vi "JSON text to Variant.vi"(6 "LVClass Serializer":refnum<class "JSONtext LVClass Serializer.lvclass">, 8 "error in (no error)":errorcluster, 9 "Data Type":variant, 10 "Offset":i32, 11 "JSON":string) -> (0 "error out":errorcluster, 1 "Variant out":variant)   [LabVIEW 2020, in "JSONtext.lvlib"]
doc: "Convert JSON to the Data Type entered, which may be a cluster or array."
uses:
  <vilib>/JDP Science/JSONtext/JSONtext.lvlib
  <vilib>/JDP Science/JSONtext/LVClass Serializer/JSONtext LVClass Serializer.lvclass
  <vilib>/Utility/Data Type/Type Definitions/Data Type.ctl
  <vilib>/JDP Science/JSONtext/support/Get String.vi
  <vilib>/JDP Science/JSONtext/support/Get Timestamp.vi
  <vilib>/JDP Science/JSONtext/support/Get I32.vi
  <vilib>/JDP Science/JSONtext/support/Coerce I32 to Variant Intger.vi
  <vilib>/JDP Science/JSONtext/support/Get I64.vi
  <vilib>/JDP Science/JSONtext/support/Get U32.vi
  <vilib>/JDP Science/JSONtext/support/Coerce U32 to Variant Intger.vi
  <vilib>/JDP Science/JSONtext/support/Get U64.vi
  <vilib>/JDP Science/JSONtext/support/Get Boolean.vi
  <vilib>/JDP Science/JSONtext/support/Get DBL.vi
  <vilib>/JDP Science/JSONtext/support/Get SGL.vi
  <vilib>/JDP Science/JSONtext/support/Unescape JSON string.vi
  <vilib>/JDP Science/JSONtext/support/quote and escape json string 2.vi
  <vilib>/JDP Science/JSONtext/support/Commas Needed.vi
  <vilib>/JDP Science/JSONtext/Parsing/Advance past whitespace and comma.vi
  <vilib>/JDP Science/JSONtext/Parsing/Advance past next JSON Value (inlined COPY).vi
  <vilib>/JDP Science/JSONtext/Parsing/Advance past Item Name.vi
  <vilib>/JDP Science/JSONtext/Base64/base64url Decode.vi
  <vilib>/JDP Science/JSONtext/Parsing/Advance past Line Ending.vi
  <vilib>/JDP Science/JSONtext/Parsing/Advance past String.vi
  <vilib>/JDP Science/JSONtext/support/Get Number Text.vi
  <vilib>/JDP Science/JSONtext/Parsing/NaN or null to Integer ERROR.vi
  <vilib>/JDP Science/JSONtext/Parsing/Advance past Number.vi
  <vilib>/Utility/error.llb/Error Cluster From Error Code.vi
  <vilib>/Utility/Data Type/Get Refnum Information.vi
  <vilib>/JDP Science/JSONtext/support/Error Cluster From Code.vi
  <vilib>/JDP Science/JDP Science Common Utilities/Timestamp/Text to Timestamp.vi
  <vilib>/Utility/Data Type/Get Numeric Information.vi
  <vilib>/JDP Science/JSONtext/Parsing/Advance past Object.vi
  <vilib>/JDP Science/JSONtext/Parsing/Parsing Error.vi
  <vilib>/Utility/Data Type/NI_Data Type.lvlib
  <vilib>/JDP Science/JDP Science Common Utilities/JDP Utility.lvlib
  <vilib>/JDP Science/JSONtext/support/Set Map/SetMap.lvlib
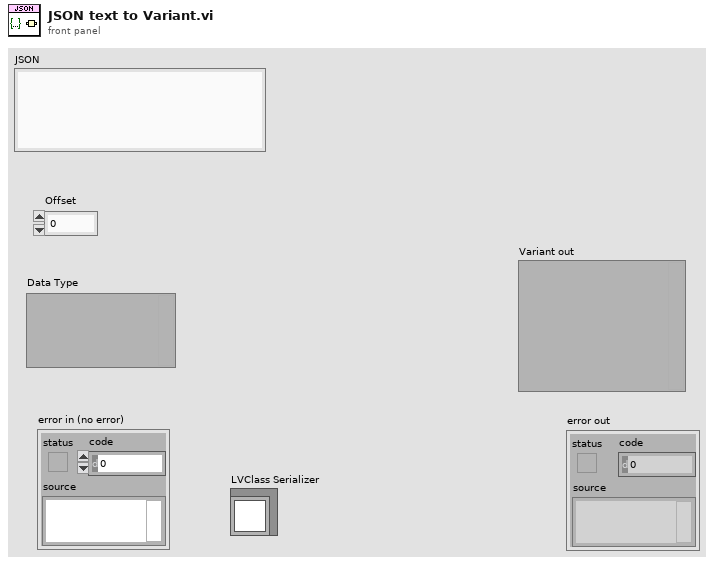
[diagram p1: front panel]
types:
  T1 = typedef "NI_Data Type.lvlib/Data Type.ctl" = enum8{"Invalid Type", "Void", "I8", "I16", "I32", "I64", "U8", "U16", "U32", "U64", "Single Float", "Double Float", "Extended Float", "Single Complex", "Double Complex", "Extended Complex", "Enum U8", "Enum U16", "Enum U32", "Enum U64", "Single Float With Unit", "Double Float With Unit", "Extended Float With Unit", "Single Complex with Unit", "Double Complex with Unit", "Extended Complex with Unit", "Boolean", "String", "Path", "Picture", "Tag", "Array", "Cluster", "Variant", "LV Variant", "Waveform", "Timestamp", "Digital Waveform", "Digital Data", "ExpressData", "Refnum", "External Data", "VI", "Poly VI", "LabVIEW Class Instance", "Fixed Point", "Set Collection", "Map Collection"}
  T2 = typedef "JSONtext.lvlib/Parsing State.ctl" = enum16{"Parser Error", "Object", "Array", "String", "Number/Other", "Leading Whitespace", "Object end", "Array end", "Value end"}
  T3 = typedef "JSONtext.lvlib/Tag Type.ctl" = enum16{"No Tag", "<JSON>", "<JOBJ>"}
  T4 = typedef "JSONtext.lvlib/JSON Value Type.ctl" = enum16{"Not a JSON Value", "JSON Object", "JSON Array", "String", "Number", "true", "false", "null"}
  T5 = typedef "JSONtext.lvlib/Found Items.ctl" = cluster{"Item offset":i32, "Offset past Item":i32, "Name offset":i32, "Offset past Name":i32, "Found":bool, "Item Type":T2, "Item Index":i32, "Start Offset":i32, "Comma Needed For Insert":T6}
  T6 = typedef "JSONtext.lvlib/Comma Needed for Insert.ctl" = enum8{"False", "True", "Following"}
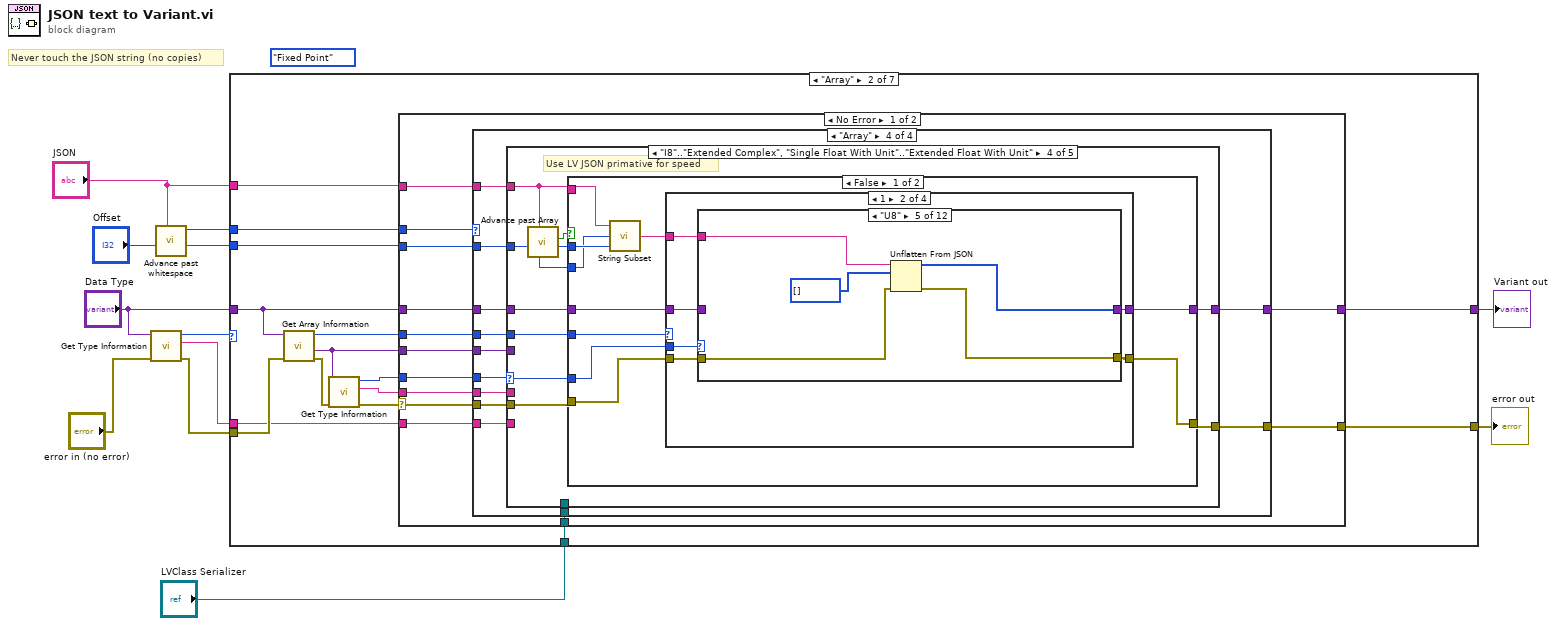
[diagram p0: block diagram]
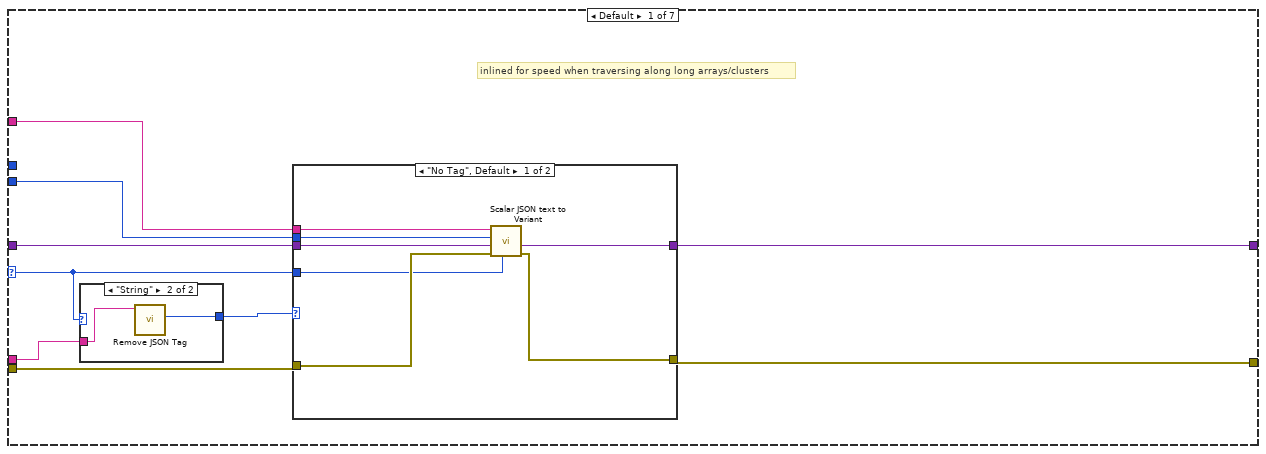
[diagram p2: hidden frame]
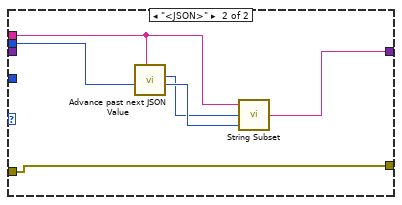
[diagram p3: hidden frame]
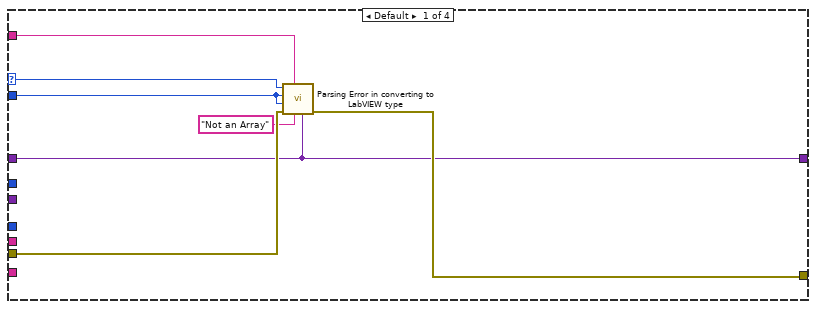
[diagram p5: hidden frame]
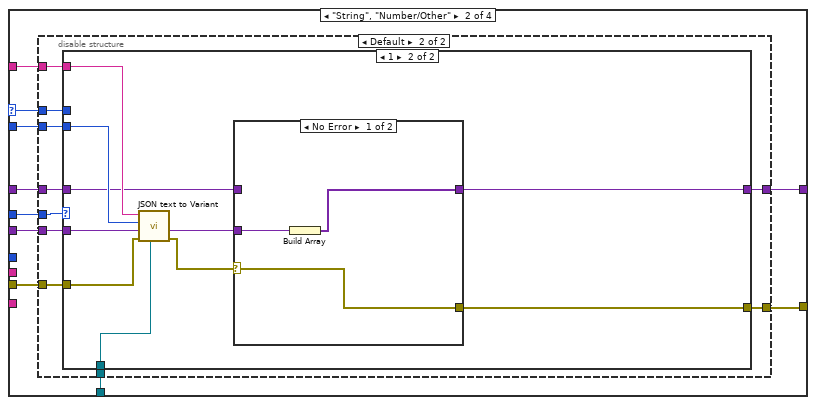
[diagram p6: hidden frame]
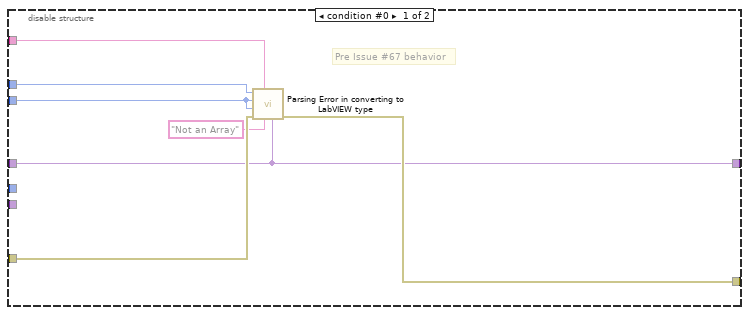
[diagram p7: hidden frame]
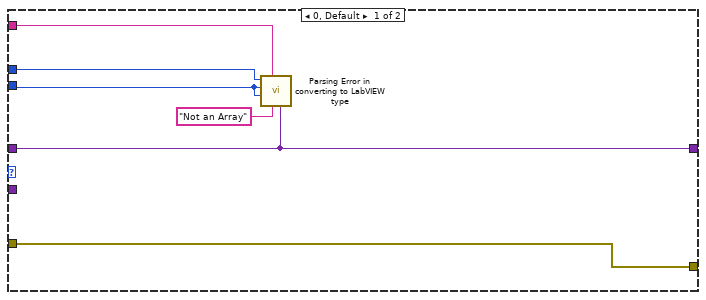
[diagram p8: hidden frame]
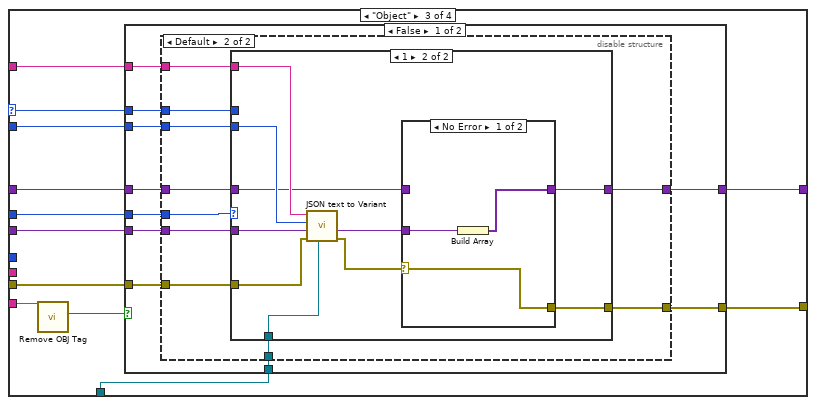
[diagram p10: hidden frame]
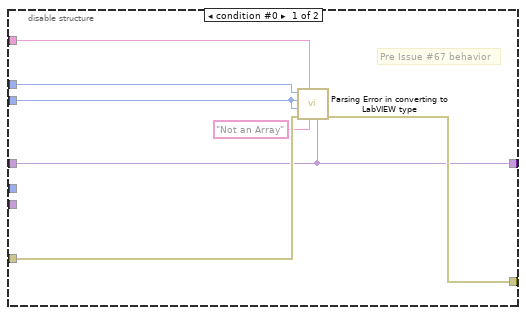
[diagram p11: hidden frame]
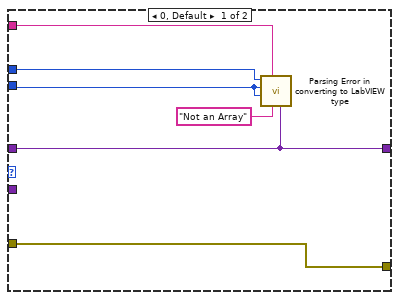
[diagram p12: hidden frame]
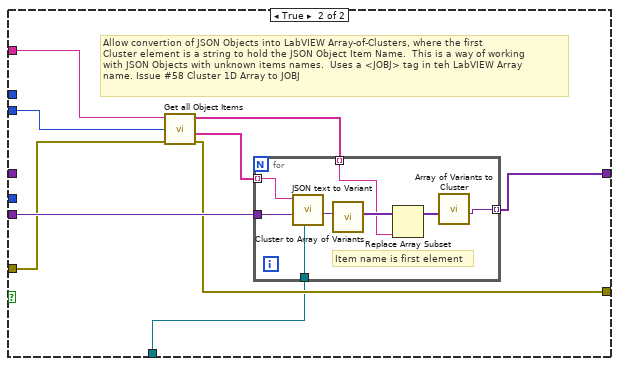
[diagram p14: hidden frame]
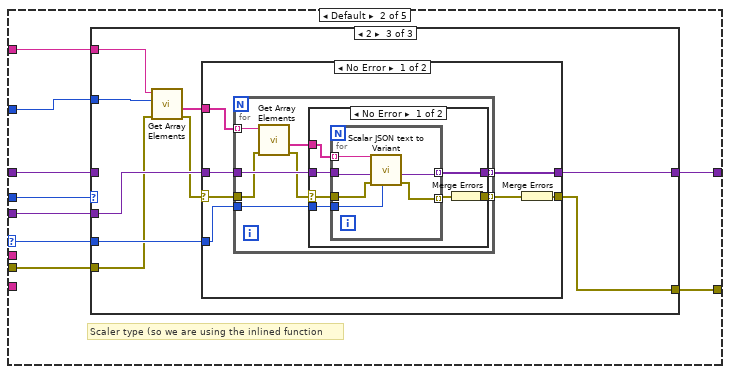
[diagram p16: hidden frame]
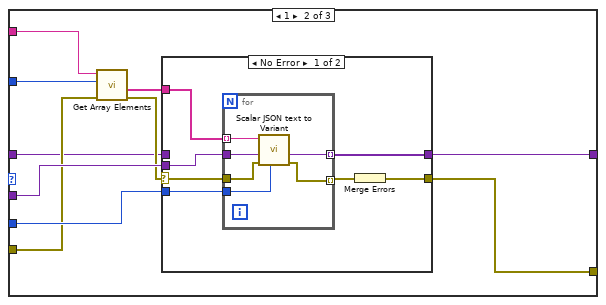
[diagram p18: hidden frame]
diagram:
  (unwired) Data_Type."Fixed Point" ("Type")
  # "Never touch the JSON string (no copies)"
  n1 = call <vilib>:"Get Type Information.vi"("error in (no error)"="error in (no error)", "variant"="Data Type") -> ("error out"=w8:errorcluster, "name"=w2:string, "type"=w12:T1)  [unwired: 5 in, 2 out]
  n2 = call <vilib>:"Advance past whitespace.vi"("JSON"="JSON", "Offset"="Offset") -> ("Offset of first non-whitespace"=w5:i32, "Parser State"=w3:T2)  [unwired: 7 in, 1 out]
  n3 = case shown="\"Array\"" w12 {
    selector: w12 -> [w14 _ _ _ _ _ w916]
    tunnel: "Data Type" -> [w21 w44 w676 w685 w885 w896 w918]
    tunnel: "JSON" -> [w19 w42 w669 w681 w880 w897 w917]
    tunnel: [w16 w48 w666 w683 w877 w890 w912] -> w9
    tunnel: w8 -> [w17 w51 w675 w684 w884 w894 w913]
    tunnel: w5 -> [w18 w40 w668 w682 w879 w889 w915]
    tunnel: [w20 w47 w659 w678 w882 w891 w914] -> w7
    tunnel: w3 -> [_ w38 _ _ _ _ _]
    tunnel: w2 -> [w15 w41 _ _ _ _ _]
    tunnel: "LVClass Serializer" -> [_ w37 w658 w677 w875 w888 w911]
    frame Default {
      # "inlined for speed when traversing along long arrays/clusters"
      n4 = case shown="\"String\"" w14 {
        tunnel: w15 -> [_ w36]
        tunnel: [_ w35] -> w13
        frame "Invalid Type", Default {
        }
        frame "String" {
          n5 = call <vilib>:"Remove JSON Tag.vi"("Name"=w36) -> ("Tag"=w35:T3)  [unwired: 9 in, 1 out]
        }
      }
      n6 = case shown="\"No Tag\", Default" w13 {
        tunnel: w21 -> [w28 _]
        tunnel: [w27 w30] -> w20
        tunnel: w19 -> [w26 w31]
        tunnel: w18 -> [w25 w34]
        tunnel: w17 -> [w24 w29]
        tunnel: [w23 w29] -> w16
        tunnel: w14 -> [w22 _]
        frame "No Tag", Default {
          n7 = call <vilib>:"Scalar JSON text to Variant.vi"("Type"=w22, "error in (no error)"=w24, "Variant (Data Type)"=w28, "Offset"=w25, "JSON"=w26) -> ("error out"=w23:errorcluster, "Variant out"=w27:variant)  [unwired: 5 in]
        }
        frame "<JSON>" {
          n8 = call <vilib>:"Advance past next JSON Value.vi"("JSON"=w31, "Offset"=w34) -> ("Offset out"=w33:i32, "Value start"=w32:i32)  [unwired: 7 in, 1 out]
          n9 = call <vilib>:"String Subset.vi"("Offset past End"=w33, "Start offset"=w32, "JSON"=w31) -> ("substring"=w30:string)  [unwired: 2 in]
        }
      }
    }
    frame "Array" {
      n10 = call <vilib>:"Get Array Information.vi"("error in (no error)"=w51, "variant"=w44) -> ("error out"=w50:errorcluster, "array element data type"=w43:variant, "number of dimensions"=w45:i32)  [unwired: 6 in, 1 out]
      n11 = call <vilib>:"Get Type Information.vi"("error in (no error)"=w50, "variant"=w43) -> ("error out"=w49:errorcluster, "name"=w39:string, "type"=w46:T1)  [unwired: 5 in, 2 out]
      n12 = case shown="No Error" w49 {
        selector: w49 -> [w64 w657]
        tunnel: [w63 w657] -> w48
        tunnel: [w62 w656] -> w47
        tunnel: w46 -> [w61 _]
        tunnel: w45 -> [w60 _]
        tunnel: w44 -> [w59 w656]
        tunnel: w43 -> [w58 _]
        tunnel: w42 -> [w57 _]
        tunnel: w41 -> [w56 _]
        tunnel: w40 -> [w55 _]
        tunnel: w39 -> [w54 _]
        tunnel: w38 -> [w53 _]
        tunnel: w37 -> [w52 _]
        frame No Error {
          n13 = case shown="\"Array\"" w53 {
            selector: w53 -> [w69 w79 w129 _]
            tunnel: w64 -> [w68 w78 w128 w208]
            tunnel: [w67 w77 w127 w207] -> w63
            tunnel: [w66 w74 w124 w206] -> w62
            tunnel: w61 -> [_ _ _ w205]
            tunnel: w60 -> [_ w73 w123 w204]
            tunnel: w59 -> [w66 w76 w126 w203]
            tunnel: w58 -> [_ w75 w125 w202]
            tunnel: w57 -> [w71 w81 w131 w201]
            tunnel: w56 -> [_ _ w121 w200]
            tunnel: w55 -> [w70 w80 w130 w199]
            tunnel: w54 -> [_ _ _ w198]
            tunnel: w52 -> [_ w72 w122 w197]
            frame Default {
              n14 = call <vilib>:"Parsing Error in converting to LabVIEW type.vi"("LV Type"=w66, "initial string"="Not an Array", "JSON"=w71, "error in (no error)"=w68, "Offset past match"=w70, "Value start"=w70, "State"=w69) -> ("error out"=w67:errorcluster)  [unwired: 4 in]
            }
            frame "String", "Number/Other" {
              n15 = disable-structure shown="Default" {
                disable-tunnel: w81 -> [w88 w97]
                disable-tunnel: w80 -> [w87 w96]
                disable-tunnel: w79 -> [w86 w90]
                disable-tunnel: w78 -> [w85 w95]
                disable-tunnel: [w84 w92] -> w77
                disable-tunnel: w76 -> [w82 w93]
                disable-tunnel: w75 -> [_ w98]
                disable-tunnel: [w82 w94] -> w74
                disable-tunnel: w73 -> [_ w91]
                disable-tunnel: w72 -> [_ w89]
                frame condition #0 {
                  # "Pre Issue #67 behavior"
                  n16 = call <vilib>:"Parsing Error in converting to LabVIEW type.vi"("LV Type"=w82, "initial string"="Not an Array", "JSON"=w88, "error in (no error)"=w85, "Offset past match"=w87, "Value start"=w87, "State"=w86) -> ("error out"=w84:errorcluster)  [unwired: 4 in]
                }
                frame condition #1 (active) {
                  n17 = case shown="1" w91 {
                    tunnel: w98 -> [_ w114]
                    tunnel: w97 -> [w103 w113]
                    tunnel: w96 -> [w101 w112]
                    tunnel: w95 -> [w99 w110]
                    tunnel: [w100 w108] -> w94
                    tunnel: w93 -> [w100 w107]
                    tunnel: [w99 w106] -> w92
                    tunnel: w90 -> [w102 _]
                    tunnel: w89 -> [_ w105]
                    frame 0, Default {
                      n18 = call <vilib>:"Parsing Error in converting to LabVIEW type.vi"("LV Type"=w100, "initial string"="Not an Array", "JSON"=w103, "Offset past match"=w101, "Value start"=w101, "State"=w102) -> ()  [unwired: 5 in, 1 out]
                    }
                    frame 1 {
                      n19 = call <vilib>:"JSON text to Variant.vi"("LVClass Serializer"=w105, "error in (no error)"=w110, "Data Type"=w114, "Offset"=w112, "JSON"=w113) -> ("error out"=w109:errorcluster, "Variant out"=w111:variant)  [unwired: 5 in]
                      n20 = case shown="No Error" w109 {
                        selector: w109 -> [w115 w118]
                        tunnel: w111 -> [w117 _]
                        tunnel: [w116 w119] -> w108
                        tunnel: w107 -> [_ w119]
                        tunnel: [w115 w118] -> w106
                        frame No Error {
                          n21 = Build Array(w117) -> (w116:variant[])
                        }
                        frame Error {
                        }
                      }
                    }
                  }
                }
              }
            }
            frame "Object" {
              n22 = call <vilib>:"Remove OBJ Tag.vi"("Name"=w121) -> ("tagged as Item Name in JSON Objects"=w120:bool)  [unwired: 9 in, 1 out]
              n23 = case shown="False" w120 {
                tunnel: w131 -> [w141 w186]
                tunnel: w130 -> [w140 w180]
                tunnel: w129 -> [w139 _]
                tunnel: w128 -> [w138 w187]
                tunnel: [w137 w184] -> w127
                tunnel: w126 -> [w136 _]
                tunnel: w125 -> [w135 w188]
                tunnel: [w134 w185] -> w124
                tunnel: w123 -> [w133 _]
                tunnel: w122 -> [w132 w183]
                frame False {
                  n24 = disable-structure shown="Default" {
                    disable-tunnel: w141 -> [w148 w157]
                    disable-tunnel: w140 -> [w147 w156]
                    disable-tunnel: w139 -> [w146 w150]
                    disable-tunnel: w138 -> [w145 w155]
                    disable-tunnel: [w144 w152] -> w137
                    disable-tunnel: w136 -> [w142 w153]
                    disable-tunnel: w135 -> [_ w158]
                    disable-tunnel: [w142 w154] -> w134
                    disable-tunnel: w133 -> [_ w151]
                    disable-tunnel: w132 -> [_ w149]
                    frame condition #0 {
                      # "Pre Issue #67 behavior"
                      n25 = call <vilib>:"Parsing Error in converting to LabVIEW type.vi"("LV Type"=w142, "initial string"="Not an Array", "JSON"=w148, "error in (no error)"=w145, "Offset past match"=w147, "Value start"=w147, "State"=w146) -> ("error out"=w144:errorcluster)  [unwired: 4 in]
                    }
                    frame condition #1 (active) {
                      n26 = case shown="1" w151 {
                        tunnel: w158 -> [_ w174]
                        tunnel: w157 -> [w163 w173]
                        tunnel: w156 -> [w161 w172]
                        tunnel: w155 -> [w159 w170]
                        tunnel: [w160 w168] -> w154
                        tunnel: w153 -> [w160 w167]
                        tunnel: [w159 w166] -> w152
                        tunnel: w150 -> [w162 _]
                        tunnel: w149 -> [_ w165]
                        frame 0, Default {
                          n27 = call <vilib>:"Parsing Error in converting to LabVIEW type.vi"("LV Type"=w160, "initial string"="Not an Array", "JSON"=w163, "Offset past match"=w161, "Value start"=w161, "State"=w162) -> ()  [unwired: 5 in, 1 out]
                        }
                        frame 1 {
                          n28 = call <vilib>:"JSON text to Variant.vi"("LVClass Serializer"=w165, "error in (no error)"=w170, "Data Type"=w174, "Offset"=w172, "JSON"=w173) -> ("error out"=w169:errorcluster, "Variant out"=w171:variant)  [unwired: 5 in]
                          n29 = case shown="No Error" w169 {
                            selector: w169 -> [w175 w178]
                            tunnel: w171 -> [w177 _]
                            tunnel: [w176 w179] -> w168
                            tunnel: w167 -> [_ w179]
                            tunnel: [w175 w178] -> w166
                            frame No Error {
                              n30 = Build Array(w177) -> (w176:variant[])
                            }
                            frame Error {
                            }
                          }
                        }
                      }
                    }
                  }
                }
                frame True {
                  # "Allow convertion of JSON Objects into LabVIEW Array-of-Clusters, where the first\nCluster element is a string to hold the JSON Object Item Name.  This is a way of working\nwith JSON Objects with unknown items names.  Uses a <JOBJ> tag in teh LabVIEW Array\nname. Issue #58 Cluster 1D Array to JOBJ"
                  n31 = call <vilib>:"Get all Object Items.vi"("error in (no error)"=w187, "Offset"=w180, "JSON"=w186) -> ("error out"=w184:errorcluster, "<JSON>"=w182:string[], "Item Names"=w181:string[])  [unwired: 5 in, 1 out]
                  n32 = for {
                    tunnel: w182 -> [w196] mode=indexing
                    tunnel: w188 -> [w195]
                    tunnel: w181 -> [w191] mode=indexing
                    tunnel: [w190] -> w185 mode=indexing
                    tunnel: w183 -> [w189]
                    # "Item name is first element"
                    n33 = call <vilib>:"JSON text to Variant.vi"("LVClass Serializer"=w189, "Data Type"=w195, "JSON"=w196) -> ("Variant out"=w193:variant)  [unwired: 7 in, 1 out]
                    n34 = call <vilib>:"Cluster to Array of Variants.vi"("Cluster"=w193) -> ("Array of Cluster Elements"=w192:variant[])  [unwired: 10 in]
                    n35 = Replace Array Subset(array=w192, new element=w191) -> (w194:variant[])  [unwired: 1 in]
                    n36 = call <vilib>:"Array of Variants to Cluster.vi"("Array of Variants"=w194) -> ("Cluster of Variants"=w190:variant)  [unwired: 10 in]
                  }
                }
              }
            }
            frame "Array" {
              n37 = case shown="\"I8\"..\"Extended Complex\", \"Single Float With Unit\"..\"Extended Float With Unit\"" w205 {
                selector: w205 -> [_ w211 _ w375 _]
                tunnel: w201 -> [_ w215 w293 w373 w593]
                tunnel: w208 -> [w209 w218 w296 w380 w592]
                tunnel: [w209 w219 w297 w379 w591] -> w207
                tunnel: [w210 w216 w294 w378 w590] -> w206
                tunnel: w204 -> [_ w214 w292 w377 w589]
                tunnel: w203 -> [w210 w213 w291 w376 w588]
                tunnel: w202 -> [_ w217 w295 _ _]
                tunnel: w199 -> [_ w212 w290 w372 w586]
                tunnel: w200 -> [_ _ w289 _ w587]
                tunnel: w198 -> [_ _ _ _ w585]
                tunnel: w197 -> [_ _ w288 _ _]
                frame "Invalid Type" {
                }
                frame Default {
                  # "Scaler type (so we are using the inlined function"
                  n38 = case shown="2" w214 {
                    tunnel: [w220 w231 w250] -> w219
                    tunnel: w218 -> [w220 w224 w248]
                    tunnel: w217 -> [_ w230 w255]
                    tunnel: [w221 w228 w253] -> w216
                    tunnel: w212 -> [_ w227 w252]
                    tunnel: w215 -> [_ w226 w251]
                    tunnel: w213 -> [w221 w222 _]
                    tunnel: w211 -> [_ w225 w249]
                    frame 0, Default {
                    }
                    frame 1 {
                      n39 = call <vilib>:"Get Array Elements.vi"("error in (no error)"=w224, "Offset"=w227, "JSON"=w226) -> ("error out"=w223:errorcluster, "<JSON>"=w229:string[])  [unwired: 6 in, 1 out]
                      n40 = case shown="No Error" w223 {
                        selector: w223 -> [w232 w245]
                        tunnel: [w237 w245] -> w231
                        tunnel: w230 -> [w236 _]
                        tunnel: w229 -> [w235 _]
                        tunnel: [w234 w246] -> w228
                        tunnel: w225 -> [w233 _]
                        tunnel: w222 -> [_ w246]
                        frame No Error {
                          n41 = for {
                            tunnel: w236 -> [w243]
                            tunnel: w232 -> [w241]
                            tunnel: [w240] -> w238 mode=indexing
                            tunnel: [w242] -> w234 mode=indexing
                            tunnel: w235 -> [w244] mode=indexing
                            tunnel: w233 -> [w239]
                            n42 = call <vilib>:"Scalar JSON text to Variant.vi"("Type"=w239, "error in (no error)"=w241, "Variant (Data Type)"=w243, "JSON"=w244) -> ("error out"=w240:errorcluster, "Variant out"=w242:variant)  [unwired: 6 in]
                          }
                          n43 = Merge Errors(w238) -> (w237:errorcluster)
                        }
                        frame Error {
                        }
                      }
                    }
                    frame 2 {
                      n44 = call <vilib>:"Get Array Elements.vi"("error in (no error)"=w248, "Offset"=w252, "JSON"=w251) -> ("error out"=w247:errorcluster, "<JSON>"=w254:string[])  [unwired: 6 in, 1 out]
                      n45 = case shown="No Error" w247 {
                        selector: w247 -> [w256 w287]
                        tunnel: w255 -> [w261 w286]
                        tunnel: w254 -> [w260 _]
                        tunnel: [w259 w286] -> w253
                        tunnel: [w258 w287] -> w250
                        tunnel: w249 -> [w257 _]
                        frame No Error {
                          n46 = for {
                            tunnel: [w270] -> w262 mode=indexing
                            tunnel: w256 -> [w264]
                            tunnel: w261 -> [w269]
                            tunnel: w260 -> [w267] mode=indexing
                            tunnel: [w268] -> w259 mode=indexing
                            tunnel: w257 -> [w265]
                            n47 = call <vilib>:"Get Array Elements.vi"("error in (no error)"=w264, "JSON"=w267) -> ("error out"=w263:errorcluster, "<JSON>"=w266:string[])  [unwired: 7 in, 1 out]
                            n48 = case shown="No Error" w263 {
                              selector: w263 -> [w271 w284]
                              tunnel: [w276 w284] -> w270
                              tunnel: w269 -> [w275 w285]
                              tunnel: [w274 w285] -> w268
                              tunnel: w266 -> [w273 _]
                              tunnel: w265 -> [w272 _]
                              frame No Error {
                                n49 = for {
                                tunnel: w275 -> [w279]
                                tunnel: w271 -> [w280]
                                tunnel: [w281] -> w277 mode=indexing
                                tunnel: [w282] -> w274 mode=indexing
                                tunnel: w273 -> [w283] mode=indexing
                                tunnel: w272 -> [w278]
                                n50 = call <vilib>:"Scalar JSON text to Variant.vi"("Type"=w278, "error in (no error)"=w280, "Variant (Data Type)"=w279, "JSON"=w283) -> ("error out"=w281:errorcluster, "Variant out"=w282:variant)  [unwired: 6 in]
                                }
                                n51 = Merge Errors(w277) -> (w276:errorcluster)
                              }
                              frame Error {
                              }
                            }
                          }
                          n52 = Merge Errors(w262) -> (w258:errorcluster)
                        }
                        frame Error {
                        }
                      }
                    }
                  }
                }
                frame "Cluster".."Waveform", "LabVIEW Class Instance".. {
                  # "Includes Sets and Maps"
                  n53 = case shown="2" w292 {
                    tunnel: [w298 w309 w329] -> w297
                    tunnel: w296 -> [w298 w308 w328]
                    tunnel: w295 -> [_ w307 w334]
                    tunnel: [w299 w306 w332] -> w294
                    tunnel: w290 -> [_ w304 w331]
                    tunnel: w293 -> [_ w305 w330]
                    tunnel: w291 -> [w299 w303 w326]
                    tunnel: w289 -> [_ _ _]
                    tunnel: w288 -> [_ w302 w325]
                    frame 0, Default {
                    }
                    frame 1 {
                      n54 = call <vilib>:"Get Array Elements.vi"("error in (no error)"=w308, "Offset"=w304, "JSON"=w305) -> ("error out"=w300:errorcluster, "<JSON>"=w301:string[])  [unwired: 6 in, 1 out]
                      n55 = case shown="No Error" w300 {
                        selector: w300 -> [w311 w324]
                        tunnel: [w315 w324] -> w309
                        tunnel: w307 -> [w314 _]
                        tunnel: [w313 w323] -> w306
                        tunnel: w301 -> [w312 _]
                        tunnel: w303 -> [_ w323]
                        tunnel: w302 -> [w310 _]
                        frame No Error {
                          n56 = for {
                            tunnel: w314 -> [w322]
                            tunnel: w311 -> [w321]
                            tunnel: [w320] -> w316 mode=indexing
                            tunnel: [w319] -> w313 mode=indexing
                            tunnel: w312 -> [w318] mode=indexing
                            tunnel: w310 -> [w317]
                            n57 = call <vilib>:"JSON text to Variant.vi"("LVClass Serializer"=w317, "error in (no error)"=w321, "Data Type"=w322, "JSON"=w318) -> ("error out"=w320:errorcluster, "Variant out"=w319:variant)  [unwired: 6 in]
                          }
                          n58 = Merge Errors(w316) -> (w315:errorcluster)
                        }
                        frame Error {
                        }
                      }
                    }
                    frame 2 {
                      n59 = call <vilib>:"Get Array Elements.vi"("error in (no error)"=w328, "Offset"=w331, "JSON"=w330) -> ("error out"=w327:errorcluster, "<JSON>"=w333:string[])  [unwired: 6 in, 1 out]
                      n60 = case shown="No Error" w327 {
                        selector: w327 -> [w337 w369]
                        tunnel: w334 -> [w341 _]
                        tunnel: w333 -> [w340 _]
                        tunnel: [w339 w368] -> w332
                        tunnel: [w338 w369] -> w329
                        tunnel: w326 -> [w336 w368]
                        tunnel: w325 -> [w335 _]
                        frame No Error {
                          n61 = for {
                            tunnel: [w351] -> w342 mode=indexing
                            tunnel: w337 -> [w346]
                            tunnel: w341 -> [w350]
                            tunnel: w340 -> [w348] mode=indexing
                            tunnel: [w349] -> w339 mode=indexing
                            tunnel: w336 -> [w344]
                            tunnel: w335 -> [w343]
                            n62 = call <vilib>:"Get Array Elements.vi"("error in (no error)"=w346, "JSON"=w348) -> ("error out"=w345:errorcluster, "<JSON>"=w347:string[])  [unwired: 7 in, 1 out]
                            n63 = case shown="No Error" w345 {
                              selector: w345 -> [w353 w367]
                              tunnel: [w357 w367] -> w351
                              tunnel: w350 -> [w356 w365]
                              tunnel: [w355 w366] -> w349
                              tunnel: w347 -> [w354 _]
                              tunnel: w344 -> [_ _]
                              tunnel: w343 -> [w352 _]
                              frame No Error {
                                n64 = for {
                                tunnel: w356 -> [w364]
                                tunnel: w353 -> [w363]
                                tunnel: [w362] -> w358 mode=indexing
                                tunnel: [w361] -> w355 mode=indexing
                                tunnel: w354 -> [w360] mode=indexing
                                tunnel: w352 -> [w359]
                                n65 = call <vilib>:"JSON text to Variant.vi"("LVClass Serializer"=w359, "error in (no error)"=w363, "Data Type"=w364, "JSON"=w360) -> ("error out"=w362:errorcluster, "Variant out"=w361:variant)  [unwired: 6 in]
                                }
                                n66 = Merge Errors(w358) -> (w357:errorcluster)
                              }
                              frame Error {
                                n67 = Build Array(w365) -> (w366:variant[])
                              }
                            }
                          }
                          n68 = Merge Errors(w342) -> (w338:errorcluster)
                        }
                        frame Error {
                        }
                      }
                    }
                  }
                }
                frame "I8".."Extended Complex", "Single Float With Unit".."Extended Float With Unit" {
                  # "Use LV JSON primative for speed"
                  n69 = call <vilib>:"Advance past Array.vi"("JSON"=w373, "Offset"=w372) -> ("Offset past Array"=w374:i32, "Empty Array"=w370:bool, "Array Start"=w371:i32)  [unwired: 6 in, 1 out]
                  n70 = case shown="False" w370 {
                    tunnel: w380 -> [w390 w583]
                    tunnel: [w389 w583] -> w379
                    tunnel: [w388 w582] -> w378
                    tunnel: w377 -> [w387 _]
                    tunnel: w376 -> [w386 w582]
                    tunnel: w375 -> [w384 _]
                    tunnel: w374 -> [w383 _]
                    tunnel: w373 -> [w382 _]
                    tunnel: w371 -> [w381 _]
                    frame False {
                      n71 = call <vilib>:"String Subset.vi"("Offset past End"=w383, "Start offset"=w381, "JSON"=w382) -> ("substring"=w385:string)  [unwired: 2 in]
                      n72 = case shown="1" w387 {
                        tunnel: w385 -> [_ w398 w461 w524]
                        tunnel: w390 -> [w391 w397 w460 w523]
                        tunnel: [w391 w396 w459 w522] -> w389
                        tunnel: [w392 w394 w457 w520] -> w388
                        tunnel: w386 -> [w392 w393 w456 w519]
                        tunnel: w384 -> [_ w395 w458 w521]
                        frame 0, Default {
                        }
                        frame 1 {
                          n73 = case shown="\"U8\"" w395 {
                            tunnel: w398 -> [_ w405 w410 w415 w420 w425 w430 w435 w440 w445 w450 w455]
                            tunnel: w397 -> [w399 w403 w408 w413 w418 w423 w428 w433 w438 w443 w448 w453]
                            tunnel: [w399 w402 w407 w412 w417 w422 w427 w432 w437 w442 w447 w452] -> w396
                            tunnel: [w400 w401 w406 w411 w416 w421 w426 w431 w436 w441 w446 w451] -> w394
                            tunnel: w393 -> [w400 _ _ _ _ _ _ _ _ _ _ _]
                            frame "Invalid Type", Default {
                            }
                            frame "Single Float", "Single Float With Unit" {
                              n74 = Unflatten From JSON(JSON string=w405, type and defaults=sgl[] [], error in (no error)=w403) -> (value=w401:sgl[], error out=w402:errorcluster)  [unwired: 4 in]
                            }
                            frame "Double Float", "Double Float With Unit" {
                              n75 = Unflatten From JSON(JSON string=w410, type and defaults=dbl[] [], error in (no error)=w408) -> (value=w406:dbl[], error out=w407:errorcluster)  [unwired: 4 in]
                            }
                            frame "Extended Float", "Extended Float With Unit" {
                              n76 = Unflatten From JSON(JSON string=w415, type and defaults=ext[] [], error in (no error)=w413) -> (value=w411:ext[], error out=w412:errorcluster)  [unwired: 4 in]
                            }
                            frame "U8" {
                              n77 = Unflatten From JSON(JSON string=w420, type and defaults=u8[] [], error in (no error)=w418) -> (value=w416:u8[], error out=w417:errorcluster)  [unwired: 4 in]
                            }
                            frame "U16" {
                              n78 = Unflatten From JSON(JSON string=w425, type and defaults=u16[] [], error in (no error)=w423) -> (value=w421:u16[], error out=w422:errorcluster)  [unwired: 4 in]
                            }
                            frame "U32" {
                              n79 = Unflatten From JSON(JSON string=w430, type and defaults=u32[] [], error in (no error)=w428) -> (value=w426:u32[], error out=w427:errorcluster)  [unwired: 4 in]
                            }
                            frame "U64" {
                              n80 = Unflatten From JSON(JSON string=w435, type and defaults=u64[] [], error in (no error)=w433) -> (value=w431:u64[], error out=w432:errorcluster)  [unwired: 4 in]
                            }
                            frame "I8" {
                              n81 = Unflatten From JSON(JSON string=w440, type and defaults=i8[] [], error in (no error)=w438) -> (value=w436:i8[], error out=w437:errorcluster)  [unwired: 4 in]
                            }
                            frame "I16" {
                              n82 = Unflatten From JSON(JSON string=w445, type and defaults=i16[] [], error in (no error)=w443) -> (value=w441:i16[], error out=w442:errorcluster)  [unwired: 4 in]
                            }
                            frame "I32" {
                              n83 = Unflatten From JSON(JSON string=w450, type and defaults=i32[] [], error in (no error)=w448) -> (value=w446:i32[], error out=w447:errorcluster)  [unwired: 4 in]
                            }
                            frame "I64" {
                              n84 = Unflatten From JSON(JSON string=w455, type and defaults=i64[] [], error in (no error)=w453) -> (value=w451:i64[], error out=w452:errorcluster)  [unwired: 4 in]
                            }
                          }
                        }
                        frame 2 {
                          n85 = case shown="\"I64\"" w458 {
                            tunnel: w461 -> [_ w468 w473 w478 w483 w488 w493 w498 w503 w508 w513 w518]
                            tunnel: w460 -> [w462 w466 w471 w476 w481 w486 w491 w496 w501 w506 w511 w516]
                            tunnel: [w462 w465 w470 w475 w480 w485 w490 w495 w500 w505 w510 w515] -> w459
                            tunnel: [w463 w464 w469 w474 w479 w484 w489 w494 w499 w504 w509 w514] -> w457
                            tunnel: w456 -> [w463 _ _ _ _ _ _ _ _ _ _ _]
                            frame "Invalid Type", Default {
                            }
                            frame "Single Float", "Single Float With Unit" {
                              n86 = Unflatten From JSON(JSON string=w468, type and defaults=sgl[][] [], error in (no error)=w466) -> (value=w464:sgl[][], error out=w465:errorcluster)  [unwired: 4 in]
                            }
                            frame "Double Float", "Double Float With Unit" {
                              n87 = Unflatten From JSON(JSON string=w473, type and defaults=dbl[][] [], error in (no error)=w471) -> (value=w469:dbl[][], error out=w470:errorcluster)  [unwired: 4 in]
                            }
                            frame "Extended Float", "Extended Float With Unit" {
                              n88 = Unflatten From JSON(JSON string=w478, type and defaults=ext[][] [], error in (no error)=w476) -> (value=w474:ext[][], error out=w475:errorcluster)  [unwired: 4 in]
                            }
                            frame "U8" {
                              n89 = Unflatten From JSON(JSON string=w483, type and defaults=u8[][] [], error in (no error)=w481) -> (value=w479:u8[][], error out=w480:errorcluster)  [unwired: 4 in]
                            }
                            frame "U16" {
                              n90 = Unflatten From JSON(JSON string=w488, type and defaults=u16[][] [], error in (no error)=w486) -> (value=w484:u16[][], error out=w485:errorcluster)  [unwired: 4 in]
                            }
                            frame "U32" {
                              n91 = Unflatten From JSON(JSON string=w493, type and defaults=u32[][] [], error in (no error)=w491) -> (value=w489:u32[][], error out=w490:errorcluster)  [unwired: 4 in]
                            }
                            frame "U64" {
                              n92 = Unflatten From JSON(JSON string=w498, type and defaults=u64[][] [], error in (no error)=w496) -> (value=w494:u64[][], error out=w495:errorcluster)  [unwired: 4 in]
                            }
                            frame "I8" {
                              n93 = Unflatten From JSON(JSON string=w503, type and defaults=i8[][] [], error in (no error)=w501) -> (value=w499:i8[][], error out=w500:errorcluster)  [unwired: 4 in]
                            }
                            frame "I16" {
                              n94 = Unflatten From JSON(JSON string=w508, type and defaults=i16[][] [], error in (no error)=w506) -> (value=w504:i16[][], error out=w505:errorcluster)  [unwired: 4 in]
                            }
                            frame "I32" {
                              n95 = Unflatten From JSON(JSON string=w513, type and defaults=i32[][] [], error in (no error)=w511) -> (value=w509:i32[][], error out=w510:errorcluster)  [unwired: 4 in]
                            }
                            frame "I64" {
                              n96 = Unflatten From JSON(JSON string=w518, type and defaults=i64[][] [], error in (no error)=w516) -> (value=w514:i64[][], error out=w515:errorcluster)  [unwired: 4 in]
                            }
                          }
                        }
                        frame 3 {
                          n97 = case shown="\"I32\"" w521 {
                            tunnel: w524 -> [_ w531 w536 w541 w546 w551 w556 w561 w566 w571 w576 w581]
                            tunnel: w523 -> [w525 w529 w534 w539 w544 w549 w554 w559 w564 w569 w574 w579]
                            tunnel: [w525 w528 w533 w538 w543 w548 w553 w558 w563 w568 w573 w578] -> w522
                            tunnel: [w526 w527 w532 w537 w542 w547 w552 w557 w562 w567 w572 w577] -> w520
                            tunnel: w519 -> [w526 _ _ _ _ _ _ _ _ _ _ _]
                            frame "Invalid Type", Default {
                            }
                            frame "Single Float", "Single Float With Unit" {
                              n98 = Unflatten From JSON(JSON string=w531, type and defaults=sgl[][][] [], error in (no error)=w529) -> (value=w527:sgl[][][], error out=w528:errorcluster)  [unwired: 4 in]
                            }
                            frame "Double Float", "Double Float With Unit" {
                              n99 = Unflatten From JSON(JSON string=w536, type and defaults=dbl[][][] [], error in (no error)=w534) -> (value=w532:dbl[][][], error out=w533:errorcluster)  [unwired: 4 in]
                            }
                            frame "Extended Float", "Extended Float With Unit" {
                              n100 = Unflatten From JSON(JSON string=w541, type and defaults=ext[][][] [], error in (no error)=w539) -> (value=w537:ext[][][], error out=w538:errorcluster)  [unwired: 4 in]
                            }
                            frame "U8" {
                              n101 = Unflatten From JSON(JSON string=w546, type and defaults=u8[][][] [], error in (no error)=w544) -> (value=w542:u8[][][], error out=w543:errorcluster)  [unwired: 4 in]
                            }
                            frame "U16" {
                              n102 = Unflatten From JSON(JSON string=w551, type and defaults=u16[][][] [], error in (no error)=w549) -> (value=w547:u16[][][], error out=w548:errorcluster)  [unwired: 4 in]
                            }
                            frame "U32" {
                              n103 = Unflatten From JSON(JSON string=w556, type and defaults=u32[][][] [], error in (no error)=w554) -> (value=w552:u32[][][], error out=w553:errorcluster)  [unwired: 4 in]
                            }
                            frame "U64" {
                              n104 = Unflatten From JSON(JSON string=w561, type and defaults=u64[][][] [], error in (no error)=w559) -> (value=w557:u64[][][], error out=w558:errorcluster)  [unwired: 4 in]
                            }
                            frame "I8" {
                              n105 = Unflatten From JSON(JSON string=w566, type and defaults=i8[][][] [], error in (no error)=w564) -> (value=w562:i8[][][], error out=w563:errorcluster)  [unwired: 4 in]
                            }
                            frame "I16" {
                              n106 = Unflatten From JSON(JSON string=w571, type and defaults=i16[][][] [], error in (no error)=w569) -> (value=w567:i16[][][], error out=w568:errorcluster)  [unwired: 4 in]
                            }
                            frame "I32" {
                              n107 = Unflatten From JSON(JSON string=w576, type and defaults=i32[][][] [], error in (no error)=w574) -> (value=w572:i32[][][], error out=w573:errorcluster)  [unwired: 4 in]
                            }
                            frame "I64" {
                              n108 = Unflatten From JSON(JSON string=w581, type and defaults=i64[][][] [], error in (no error)=w579) -> (value=w577:i64[][][], error out=w578:errorcluster)  [unwired: 4 in]
                            }
                          }
                        }
                      }
                    }
                    frame True {
                    }
                  }
                }
                frame "String" {
                  n109 = call <vilib>:"JSON Tags on Array.vi"("Array Name"=w587, "Element Name"=w585) -> ("Tag"=w584:T3)  [unwired: 9 in]
                  n110 = case shown="\"No Tag\", Default" w584 {
                    tunnel: w593 -> [w600 w637]
                    tunnel: w592 -> [w599 w636]
                    tunnel: [w598 w635] -> w591
                    tunnel: [w597 w634] -> w590
                    tunnel: w589 -> [w596 w633]
                    tunnel: w588 -> [w595 w632]
                    tunnel: w586 -> [w594 w631]
                    frame "No Tag", Default {
                      # "#ds issue #2 Can't use LV primative\nbecause it mishandles zero bytes."
                      n111 = case shown="1" w596 {
                        tunnel: w600 -> [_ w607 w615]
                        tunnel: w599 -> [w601 w604 w616]
                        tunnel: [w601 w605 w617] -> w598
                        tunnel: [w602 w606 w618] -> w597
                        tunnel: w595 -> [w602 _ _]
                        tunnel: w594 -> [_ w603 w614]
                        frame 0, Default {
                        }
                        frame 1 {
                          n112 = call <vilib>:"Get Array Elements.vi"("error in (no error)"=w604, "Offset"=w603, "JSON"=w607) -> ("error out"=w609:errorcluster, "<JSON>"=w608:string[])  [unwired: 6 in, 1 out]
                          n113 = for {
                            tunnel: w608 -> [w613] mode=indexing
                            tunnel: [w612] -> w606 mode=indexing
                            shift-right: [w611] -> w605
                            shift-left: w609 -> [w610]
                            n114 = call <vilib>:"Strip Quotes and Unescape.vi"("error in (no error)"=w610, "String"=w613) -> ("error out"=w611:errorcluster, "result string"=w612:string)  [unwired: 8 in]
                          }
                        }
                        frame 2 {
                          n115 = call <vilib>:"Get Array Elements.vi"("error in (no error)"=w616, "Offset"=w614, "JSON"=w615) -> ("error out"=w620:errorcluster, "<JSON>"=w619:string[])  [unwired: 6 in, 1 out]
                          n116 = for {
                            tunnel: w619 -> [w626] mode=indexing
                            tunnel: [w623] -> w618 mode=indexing
                            shift-right: [w622] -> w617
                            shift-left: w620 -> [w625]
                            n117 = call <vilib>:"Get Array Elements.vi"("error in (no error)"=w625, "JSON"=w626) -> ("error out"=w621:errorcluster, "<JSON>"=w624:string[])  [unwired: 7 in, 1 out]
                            n118 = for {
                              tunnel: w624 -> [w630] mode=indexing
                              tunnel: [w629] -> w623 mode=indexing
                              shift-right: [w628] -> w622
                              shift-left: w621 -> [w627]
                              n119 = call <vilib>:"Strip Quotes and Unescape.vi"("error in (no error)"=w627, "String"=w630) -> ("error out"=w628:errorcluster, "result string"=w629:string)  [unwired: 8 in]
                            }
                          }
                        }
                      }
                    }
                    frame "<JSON>" {
                      # "JSON text"
                      n120 = case shown="2" w633 {
                        tunnel: w637 -> [_ w644 w646]
                        tunnel: w636 -> [w638 w643 w647]
                        tunnel: [w638 w642 w648] -> w635
                        tunnel: [w639 w641 w649] -> w634
                        tunnel: w632 -> [w639 _ _]
                        tunnel: w631 -> [_ w640 w645]
                        frame 0, Default {
                        }
                        frame 1 {
                          n121 = call <vilib>:"Get Array Elements.vi"("error in (no error)"=w643, "Offset"=w640, "JSON"=w644) -> ("error out"=w642:errorcluster, "<JSON>"=w641:string[])  [unwired: 6 in, 1 out]
                        }
                        frame 2 {
                          n122 = call <vilib>:"Get Array Elements.vi"("error in (no error)"=w647, "Offset"=w645, "JSON"=w646) -> ("error out"=w651:errorcluster, "<JSON>"=w650:string[])  [unwired: 6 in, 1 out]
                          n123 = for {
                            tunnel: w650 -> [w655] mode=indexing
                            tunnel: [w652] -> w649 mode=indexing
                            shift-right: [w653] -> w648
                            shift-left: w651 -> [w654]
                            n124 = call <vilib>:"Get Array Elements.vi"("error in (no error)"=w654, "JSON"=w655) -> ("error out"=w653:errorcluster, "<JSON>"=w652:string[])  [unwired: 7 in, 1 out]
                          }
                        }
                      }
                    }
                  }
                }
              }
            }
          }
        }
        frame Error {
        }
      }
    }
    frame "Waveform" {
      # "Attributes not supported"
      n125 = Variant To Data(error in=w675, type=waveform(dbl) {"t0"=timestamp(0 s since 1904-01-01), "dt"=1.0, "Y"=[]} ("waveform"), Variant=w676) -> (data=w673:waveform(dbl), error out=w667:errorcluster)
      n126 = Unbundle By Name(w673) -> ("t0"=w672:timestamp, "dt"=w671:dbl, "Y"=w670:dbl[])  [unwired: 1 out]
      n127 = Bundle("t0"=w672, "dt"=w671, "Y"=w670) -> (w664:cluster{"t0":timestamp, "dt":dbl, "Y":dbl[]})  [unwired: 1 in]
      n128 = call <vilib>:"JSON text to Variant.vi"("LVClass Serializer"=w658, "error in (no error)"=w667, "Data Type"=w664, "Offset"=w668, "JSON"=w669) -> ("error out"=w666:errorcluster, "Variant out"=w665:variant)  [unwired: 5 in]
      n129 = Variant To Data(type=w664, Variant=w665) -> (data=w663:cluster{"t0":timestamp, "dt":dbl, "Y":dbl[]})  [unwired: 1 in, 1 out]
      n130 = Unbundle By Name(w663) -> ("t0"=w662:timestamp, "dt"=w661:dbl, "Y"=w660:dbl[])
      n131 = Bundle By Name("t0"=w662, "dt"=w661, "Y"=w660) -> (w659:waveform(dbl))  [unwired: 1 in]
    }
    frame "Cluster" {
      n132 = call <vilib>:"JSON type.vi"("Offset"=w682, "JSON"=w681) -> ("Item Offset"=w680:i32, "JSON Value Type"=w679:T4)  [unwired: 8 in]
      n133 = case shown="\"JSON Object\"" w679 {
        selector: w679 -> [w690 _ w804]
        tunnel: w685 -> [w687 w711 w814]
        tunnel: w684 -> [w686 w709 w812]
        tunnel: [w687 w698 w805] -> w678
        tunnel: [w688 w707 w811] -> w683
        tunnel: w681 -> [_ w704 w808]
        tunnel: w680 -> [_ w703 w807]
        tunnel: w677 -> [_ w693 w803]
        frame Default {
          # "Issue #65"
          n134 = Format Into String(w690) -> (resulting string=w689:string)  [unwired: 3 in, 1 out]
          n135 = call <vilib>:"Format Error.vi"("error code (402842)"=402844, "error in (no error)"=w686, "message part 2"=w689, "error message"="Cannot Get as a Cluster: " ("format string")) -> ("error out"=w688:errorcluster)  [unwired: 7 in]
        }
        frame "JSON Object" {
          n136 = Variant To Data(error in=w709, type=variant[] [], Variant=w711) -> (data=w705:variant[], error out=w706:errorcluster)
          n137 = for {
            tunnel: w705 -> [w798] mode=indexing
            tunnel: w706 -> [w797]
            tunnel: [w796] -> w702 mode=indexing
            tunnel: [w794] -> w699 mode=indexing
            tunnel: [w795] -> w701 mode=indexing
            tunnel: [w792] -> w700 mode=indexing
            n138 = call <vilib>:"Get Type Information.vi"("error in (no error)"=w797, "variant"=w798) -> ("error out"=w796:errorcluster, "name"=w793:string, "type"=w794:T1)  [unwired: 5 in, 2 out]
            n139 = case shown="\"String\", \"Array\"" w794 {
              tunnel: w793 -> [w799 w802]
              tunnel: [_ w801] -> w795
              tunnel: [w799 w800] -> w791
              frame Default {
              }
              frame "String", "Array" {
                n140 = call <vilib>:"Remove JSON Tag.vi"("Name"=w802) -> ("Tag"=w801:T3, "Name (tag stripped)"=w800:string)  [unwired: 9 in]
              }
            }
            n141 = call <vilib>:"Quote and Escape JSON string.vi"("Plain Text"=w791) -> ("<JSON>"=w792:string)  [unwired: 10 in]
          }
          n142 = call <vilib>:"Find Object Item Locations by Names.vi"("Insertion point if not found"=TRUE, "Item Names <JSON>"=w700, "error in (no error)"=w706, "Object Offset"=w703, "JSON"=w704) -> ("error out"=w694:errorcluster, "Items"=w696:T5[])  [unwired: 5 in]
          n143 = case shown="No Error" w694 {
            tunnel: [w720 w789] -> w697
            tunnel: [w719 w790] -> w708
            tunnel: w702 -> [w718 w789]
            tunnel: w696 -> [w717 _]
            tunnel: w701 -> [w716 _]
            tunnel: w699 -> [w715 _]
            tunnel: w705 -> [w714 w790]
            tunnel: w704 -> [w713 _]
            tunnel: w693 -> [w712 _]
            frame No Error {
              n144 = for {
                tunnel: w714 -> [w732] mode=indexing
                tunnel: w713 -> [w731]
                tunnel: [w730] -> w720 mode=indexing
                tunnel: [w729] -> w719 mode=indexing
                tunnel: w718 -> [w728] mode=indexing
                tunnel: w715 -> [w727] mode=indexing
                tunnel: w717 -> [w726] mode=indexing
                tunnel: w716 -> [w722] mode=indexing
                tunnel: w712 -> [w721]
                n145 = Unbundle By Name(w726) -> ("Found"=w725:bool, "Item offset"=w724:i32, "Offset past Item"=w723:i32)
                n146 = case shown="True" w725 {
                  tunnel: w731 -> [_ w744]
                  tunnel: w724 -> [_ w743]
                  tunnel: w732 -> [w734 w742]
                  tunnel: [w734 w738] -> w729
                  tunnel: w728 -> [w733 w741]
                  tunnel: [w733 w740] -> w730
                  tunnel: w727 -> [_ w739]
                  tunnel: w723 -> [_ w736]
                  tunnel: w722 -> [_ w737]
                  tunnel: w721 -> [_ w735]
                  frame False {
                  }
                  frame True {
                    n147 = case shown="\"No Tag\", Default" w737 {
                      tunnel: w744 -> [w753 w776]
                      tunnel: w743 -> [w752 w775]
                      tunnel: w742 -> [w751 w769]
                      tunnel: w741 -> [w750 w771]
                      tunnel: [w749 w770] -> w740
                      tunnel: w739 -> [w746 w772]
                      tunnel: [w748 w773] -> w738
                      tunnel: w736 -> [_ w774]
                      tunnel: w735 -> [w745 w768]
                      frame "No Tag", Default {
                        n148 = call <vilib>:"Is Scaler Type.vi"("Type"=w746) -> ("Scaler Type"=w747:bool)  [unwired: 2 in]
                        n149 = case shown="False" w747 {
                          tunnel: w753 -> [w760 w767]
                          tunnel: w752 -> [w759 w766]
                          tunnel: [w758 w765] -> w748
                          tunnel: w751 -> [w756 w764]
                          tunnel: w750 -> [w755 w763]
                          tunnel: [w757 w762] -> w749
                          tunnel: w746 -> [w754 _]
                          tunnel: w745 -> [_ w761]
                          frame True {
                            n150 = call <vilib>:"Scalar JSON text to Variant.vi"("Type"=w754, "error in (no error)"=w755, "Variant (Data Type)"=w756, "Offset"=w759, "JSON"=w760) -> ("error out"=w757:errorcluster, "Variant out"=w758:variant)  [unwired: 5 in]
                          }
                          frame False {
                            n151 = call <vilib>:"JSON text to Variant.vi"("LVClass Serializer"=w761, "error in (no error)"=w763, "Data Type"=w764, "Offset"=w766, "JSON"=w767) -> ("error out"=w762:errorcluster, "Variant out"=w765:variant)  [unwired: 5 in]
                          }
                        }
                      }
                      frame "<JSON>" {
                        # "<JSON>"
                        n152 = case shown="\"Array\"" w772 {
                          tunnel: w776 -> [w783 w788]
                          tunnel: w775 -> [w782 w787]
                          tunnel: w774 -> [_ w786]
                          tunnel: [w779 w785] -> w773
                          tunnel: w771 -> [w780 w784]
                          tunnel: [w778 w784] -> w770
                          tunnel: w769 -> [w781 _]
                          tunnel: w768 -> [w777 _]
                          frame "Array" {
                            n153 = call <vilib>:"JSON text to Variant.vi"("LVClass Serializer"=w777, "error in (no error)"=w780, "Data Type"=w781, "Offset"=w782, "JSON"=w783) -> ("error out"=w778:errorcluster, "Variant out"=w779:variant)  [unwired: 5 in]
                          }
                          frame "String", Default {
                            n154 = call <vilib>:"String Subset.vi"("Offset past End"=w786, "Start offset"=w787, "JSON"=w788) -> ("substring"=w785:string)  [unwired: 2 in]
                          }
                        }
                      }
                    }
                  }
                }
              }
            }
            frame Error {
              # "Issue 40"
            }
          }
          n155 = call <vilib>:"Array of Variants to Cluster.vi"("Array of Variants"=w708) -> ("Cluster of Variants"=w698:variant)  [unwired: 10 in]
          n156 = Merge Errors(w694, w697) -> (w707:errorcluster)
        }
        frame "JSON Array" {
          n157 = Variant To Data(error in=w812, type=variant[] [], Variant=w814) -> (data=w809:variant[], error out=w810:errorcluster)
          n158 = call <vilib>:"Possible Ragged Array.vi"("Array"=w809) -> ("Ragged Array posible"=w806:bool)  [unwired: 10 in]
          n159 = case shown="True" w806 {
            tunnel: [w828 w868] -> w811
            tunnel: w807 -> [w816 w871]
            tunnel: w810 -> [w827 w869]
            tunnel: w809 -> [w820 w874]
            tunnel: w808 -> [w819 w872]
            tunnel: [w817 w866] -> w805
            tunnel: w804 -> [w826 _]
            tunnel: w803 -> [w815 w865]
            frame False {
              # "First Cluster Element Unnamed"
              n160 = Index Array(array=w820) -> (element=w825:variant)  [unwired: 1 in]
              n161 = call <vilib>:"Get Type Information.vi"("variant"=w825) -> ("name"=w822:string, "type"=w823:T1)  [unwired: 6 in, 3 out]
              n162 = case shown="\"String\", \"Array\"" w823 {
                tunnel: w822 -> [w829 w831]
                tunnel: [w829 w830] -> w824
                frame Default {
                }
                frame "String", "Array" {
                  n163 = call <vilib>:"Remove JSON Tag.vi"("Name"=w831) -> ("Name (tag stripped)"=w830:string)  [unwired: 9 in, 1 out]
                }
              }
              n164 = Empty String/Path?(string/path=w824) -> (empty?=w821:bool)
              n165 = case shown="True" w821 {
                tunnel: [w835 w846] -> w828
                tunnel: w827 -> [w834 w841]
                tunnel: w826 -> [w833 _]
                tunnel: [w832 w843] -> w818
                tunnel: w820 -> [w832 w845]
                tunnel: w819 -> [_ w844]
                tunnel: w816 -> [_ w842]
                tunnel: w815 -> [_ w839]
                frame False {
                  n166 = Format Into String(w833) -> (resulting string=w836:string)  [unwired: 3 in, 1 out]
                  n167 = call <vilib>:"Format Error.vi"("error code (402842)"=402844, "error in (no error)"=w834, "message part 2"=w836, "error message"="Cannot Get Array as a Cluster: " ("format string")) -> ("error out"=w835:errorcluster)  [unwired: 7 in]
                }
                frame True {
                  # "Unnamed cluster elements\n--> JSON Array"
                  n168 = call <vilib>:"Get Array Elements.vi"("error in (no error)"=w841, "Offset"=w842, "JSON"=w844) -> ("error out"=w840:errorcluster, "<JSON>"=w847:string[])  [unwired: 6 in, 1 out]
                  n169 = for {
                    tunnel: w845 -> [w856] mode=indexing
                    tunnel: w840 -> [w854]
                    tunnel: [w853] -> w848 mode=indexing
                    tunnel: [w855] -> w843 mode=indexing
                    tunnel: w847 -> [w852]
                    tunnel: w839 -> [w849]
                    i -> [w850]
                    n170 = Index Array(array=w852, index=w850) -> (element=w851:string)
                    n171 = case shown="Default" w851 {
                      selector: w851 -> [_ w860]
                      tunnel: w856 -> [w858 w864]
                      tunnel: [w858 w863] -> w855
                      tunnel: w854 -> [w857 w862]
                      tunnel: [w857 w861] -> w853
                      tunnel: w849 -> [_ w859]
                      frame "" {
                      }
                      frame Default {
                        n172 = call <vilib>:"JSON text to Variant.vi"("LVClass Serializer"=w859, "error in (no error)"=w862, "Data Type"=w864, "JSON"=w860) -> ("error out"=w861:errorcluster, "Variant out"=w863:variant)  [unwired: 6 in]
                      }
                    }
                  }
                  n173 = Merge Errors(w848) -> (w846:errorcluster)
                }
              }
              n174 = call <vilib>:"Array of Variants to Cluster.vi"("Array of Variants"=w818) -> ("Cluster of Variants"=w817:variant)  [unwired: 10 in]
            }
            frame True {
              # "Let a JSON Array be valid for an Array as sole element in a Cluster, as this is a way of doing \"Ragged\" arrays in LabVIEW."
              n175 = Index Array(array=w874) -> (element=w873:variant)  [unwired: 1 in]
              n176 = call <vilib>:"JSON text to Variant.vi"("LVClass Serializer"=w865, "error in (no error)"=w869, "Data Type"=w873, "Offset"=w871, "JSON"=w872) -> ("error out"=w868:errorcluster, "Variant out"=w870:variant)  [unwired: 5 in]
              n177 = Build Array(w870) -> (w867:variant[])
              n178 = call <vilib>:"Array of Variants to Cluster.vi"("Array of Variants"=w867) -> ("Cluster of Variants"=w866:variant)  [unwired: 10 in]
            }
          }
        }
      }
    }
    frame "Variant", "LV Variant" {
      # "Unwrap and rewrap"
      n179 = Variant To Data(error in=w884, type=variant, Variant=w885) -> (data=w876:variant, error out=w881:errorcluster)
      n180 = call <vilib>:"JSON text to Variant.vi"("LVClass Serializer"=w875, "error in (no error)"=w881, "Data Type"=w876, "Offset"=w879, "JSON"=w880) -> ("error out"=w877:errorcluster, "Variant out"=w878:variant)  [unwired: 5 in]
      n181 = To Variant(anything=w878) -> (Variant=w882:variant)
    }
    frame "LabVIEW Class Instance" {
      n182 = Variant To Data(error in=w894, type=refnum<class> refnum ("LabVIEW Object"), Variant=w896) -> (data=w892:refnum<class>, error out=w895:errorcluster)
      n183 = Not Equal?(x=w888, y=refnum<class "JSONtext LVClass Serializer.lvclass"> refnum) -> (x != y?=w886:bool)
      n184 = case shown="False" w886 {
        tunnel: w888 -> [_ w910]
        tunnel: w897 -> [w903 w909]
        tunnel: w895 -> [w899 w908]
        tunnel: w892 -> [w898 w907]
        tunnel: [w901 w906] -> w891
        tunnel: [w900 w905] -> w890
        tunnel: w889 -> [w902 w904]
        frame False {
          n185 = call <vilib>:"JSON to LVObject.vi"("error in (no error)"=w899, "JSON"=w903, "Offset of first non-whitespace"=w902, "LabVIEW Object in"=w898) -> ("error out"=w900:errorcluster, "LabVIEW Object out"=w901:refnum<class>)  [unwired: 6 in]
        }
        frame True {
          # "Issue #56 Way of providing alternate format\nof LVObjects"
          n186 = call-dynamic <vilib>:"JSON to LVObject.vi"("JSONtext LVClass Serializer in"=w910, "error in (no error)"=w908, "Object Type"=w907, "Offset"=w904, "JSON"=w909) -> ("error out"=w905:errorcluster, "Object"=w906:refnum<class>)  [unwired: 5 in]
        }
      }
    }
    frame "Fixed Point".. {
      n187 = Type Cast(type=u8 0, x=w916) -> (*(type *) &x=w919:u8)
      n188 = case shown="46" w919 {
        tunnel: w918 -> [w922 w929 w932 w939]
        tunnel: w917 -> [_ w928 w934 w941]
        tunnel: w916 -> [_ w927 _ _]
        tunnel: w915 -> [_ w926 w930 w938]
        tunnel: [w922 w925 w931 w937] -> w914
        tunnel: w913 -> [w921 w924 w936 w943]
        tunnel: [w921 w923 w935 w942] -> w912
        tunnel: w911 -> [_ _ w933 w940]
        frame 0, Default {
        }
        frame 45 {
          # "Fixed Point"
          n189 = call <vilib>:"Scalar JSON text to Variant.vi"("Type"=w927, "error in (no error)"=w924, "Variant (Data Type)"=w929, "Offset"=w926, "JSON"=w928) -> ("error out"=w923:errorcluster, "Variant out"=w925:variant)  [unwired: 5 in]
        }
        frame 46 {
          # "46 == Set in LabVIEW 2019 and later\nIssue #74"
          n190 = call <vilib>:"JSON To Set.vi"("LVClass Serializer"=w933, "error in (no error)"=w936, "Set Type"=w932, "Offset"=w930, "<JSON>"=w934) -> ("error out"=w935:errorcluster, "Set"=w931:variant)  [unwired: 5 in]
        }
        frame 47 {
          # "47 == Map in LabVIEW 2019 and later\nIssue #74"
          n191 = call <vilib>:"JSON to Map.vi"("LVClass Serializer"=w940, "error in (no error)"=w943, "Map Type in"=w939, "Offset"=w938, "<JSON>"=w941) -> ("error out"=w942:errorcluster, "Map"=w937:variant)  [unwired: 5 in]
        }
      }
    }
  }
  "Variant out" <- w7
  "error out" <- w9
